vi "UI_updatePuzzle.vi"(8 "error in (no error)":errorcluster, 10 "Puzzle":refnum<vi>, 11 "Puzzle state":string) -> (0 "error out":errorcluster)   [LabVIEW 2020]
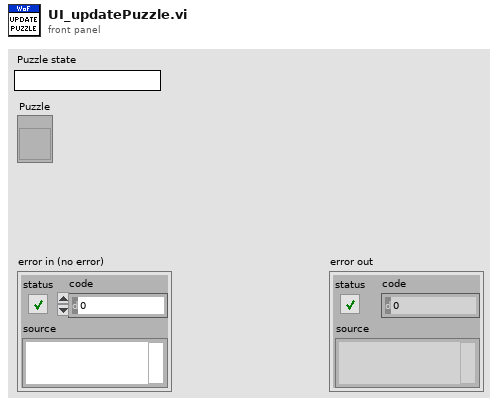
[diagram p1: front panel]
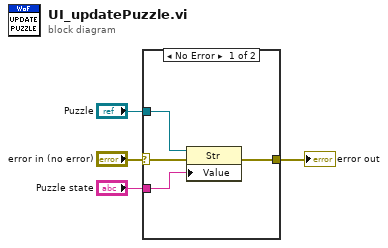
[diagram p0: block diagram]
diagram:
  n1 = case shown="No Error" "error in (no error)" {
    selector: "error in (no error)" -> [w8 w9]
    tunnel: [w5 w9] -> w3
    tunnel: "Puzzle state" -> [w6 _]
    tunnel: "Puzzle" -> [w7 _]
    frame No Error {
      n2 = property class="Str"(reference=w7, error in=w8, "Value"=w6) -> (error out=w5:errorcluster)  [unwired: 1 out]
    }
    frame Error {
    }
  }
  "error out" <- w3
